vi "Plots_testing.vi"() -> ()   [LabVIEW 2016]
uses:
  <vilib>/Heliosphere Research LLC/Advanced Plotting Toolkit/api_plotting/Histogram2DProperties.ctl
  <vilib>/Heliosphere Research LLC/Advanced Plotting Toolkit/properties/Colormap.ctl
  <vilib>/Heliosphere Research LLC/Advanced Plotting Toolkit/properties/Colormap_Map.ctl
  <vilib>/Heliosphere Research LLC/Advanced Plotting Toolkit/properties/Colormap_Scaling.ctl
  <vilib>/Heliosphere Research LLC/Advanced Plotting Toolkit/properties/Display.ctl
  <vilib>/Heliosphere Research LLC/Advanced Plotting Toolkit/api_core/NewPlotType.ctl
  <vilib>/Heliosphere Research LLC/Advanced Plotting Toolkit/api_plotting/ArrayViewProperties.ctl
  SubVi's/SW_Globals.vi
  <vilib>/Heliosphere Research LLC/Advanced Plotting Toolkit/api_plotting/Histogram2D_Automatic.vi
  <vilib>/Heliosphere Research LLC/Advanced Plotting Toolkit/Advanced Plotting Toolkit.lvlib
panel:
  out "Picture 2":picture
  in  "Properties":T1={"Normalize"=FALSE, "Colormap"={"Map"=enum."Automatic", "Value Min"=nan, "Value Max"=nan, "Scaling"=enum."Default", "Reverse"=FALSE}, "Display"={"Alpha"=nan, "Z Order"=nan}}
  out "Count":u32[](array[numeric])
  out "X coords":i32[](array[numeric])
  out "Y coords":i32[](array[numeric])
  out "Picture":picture
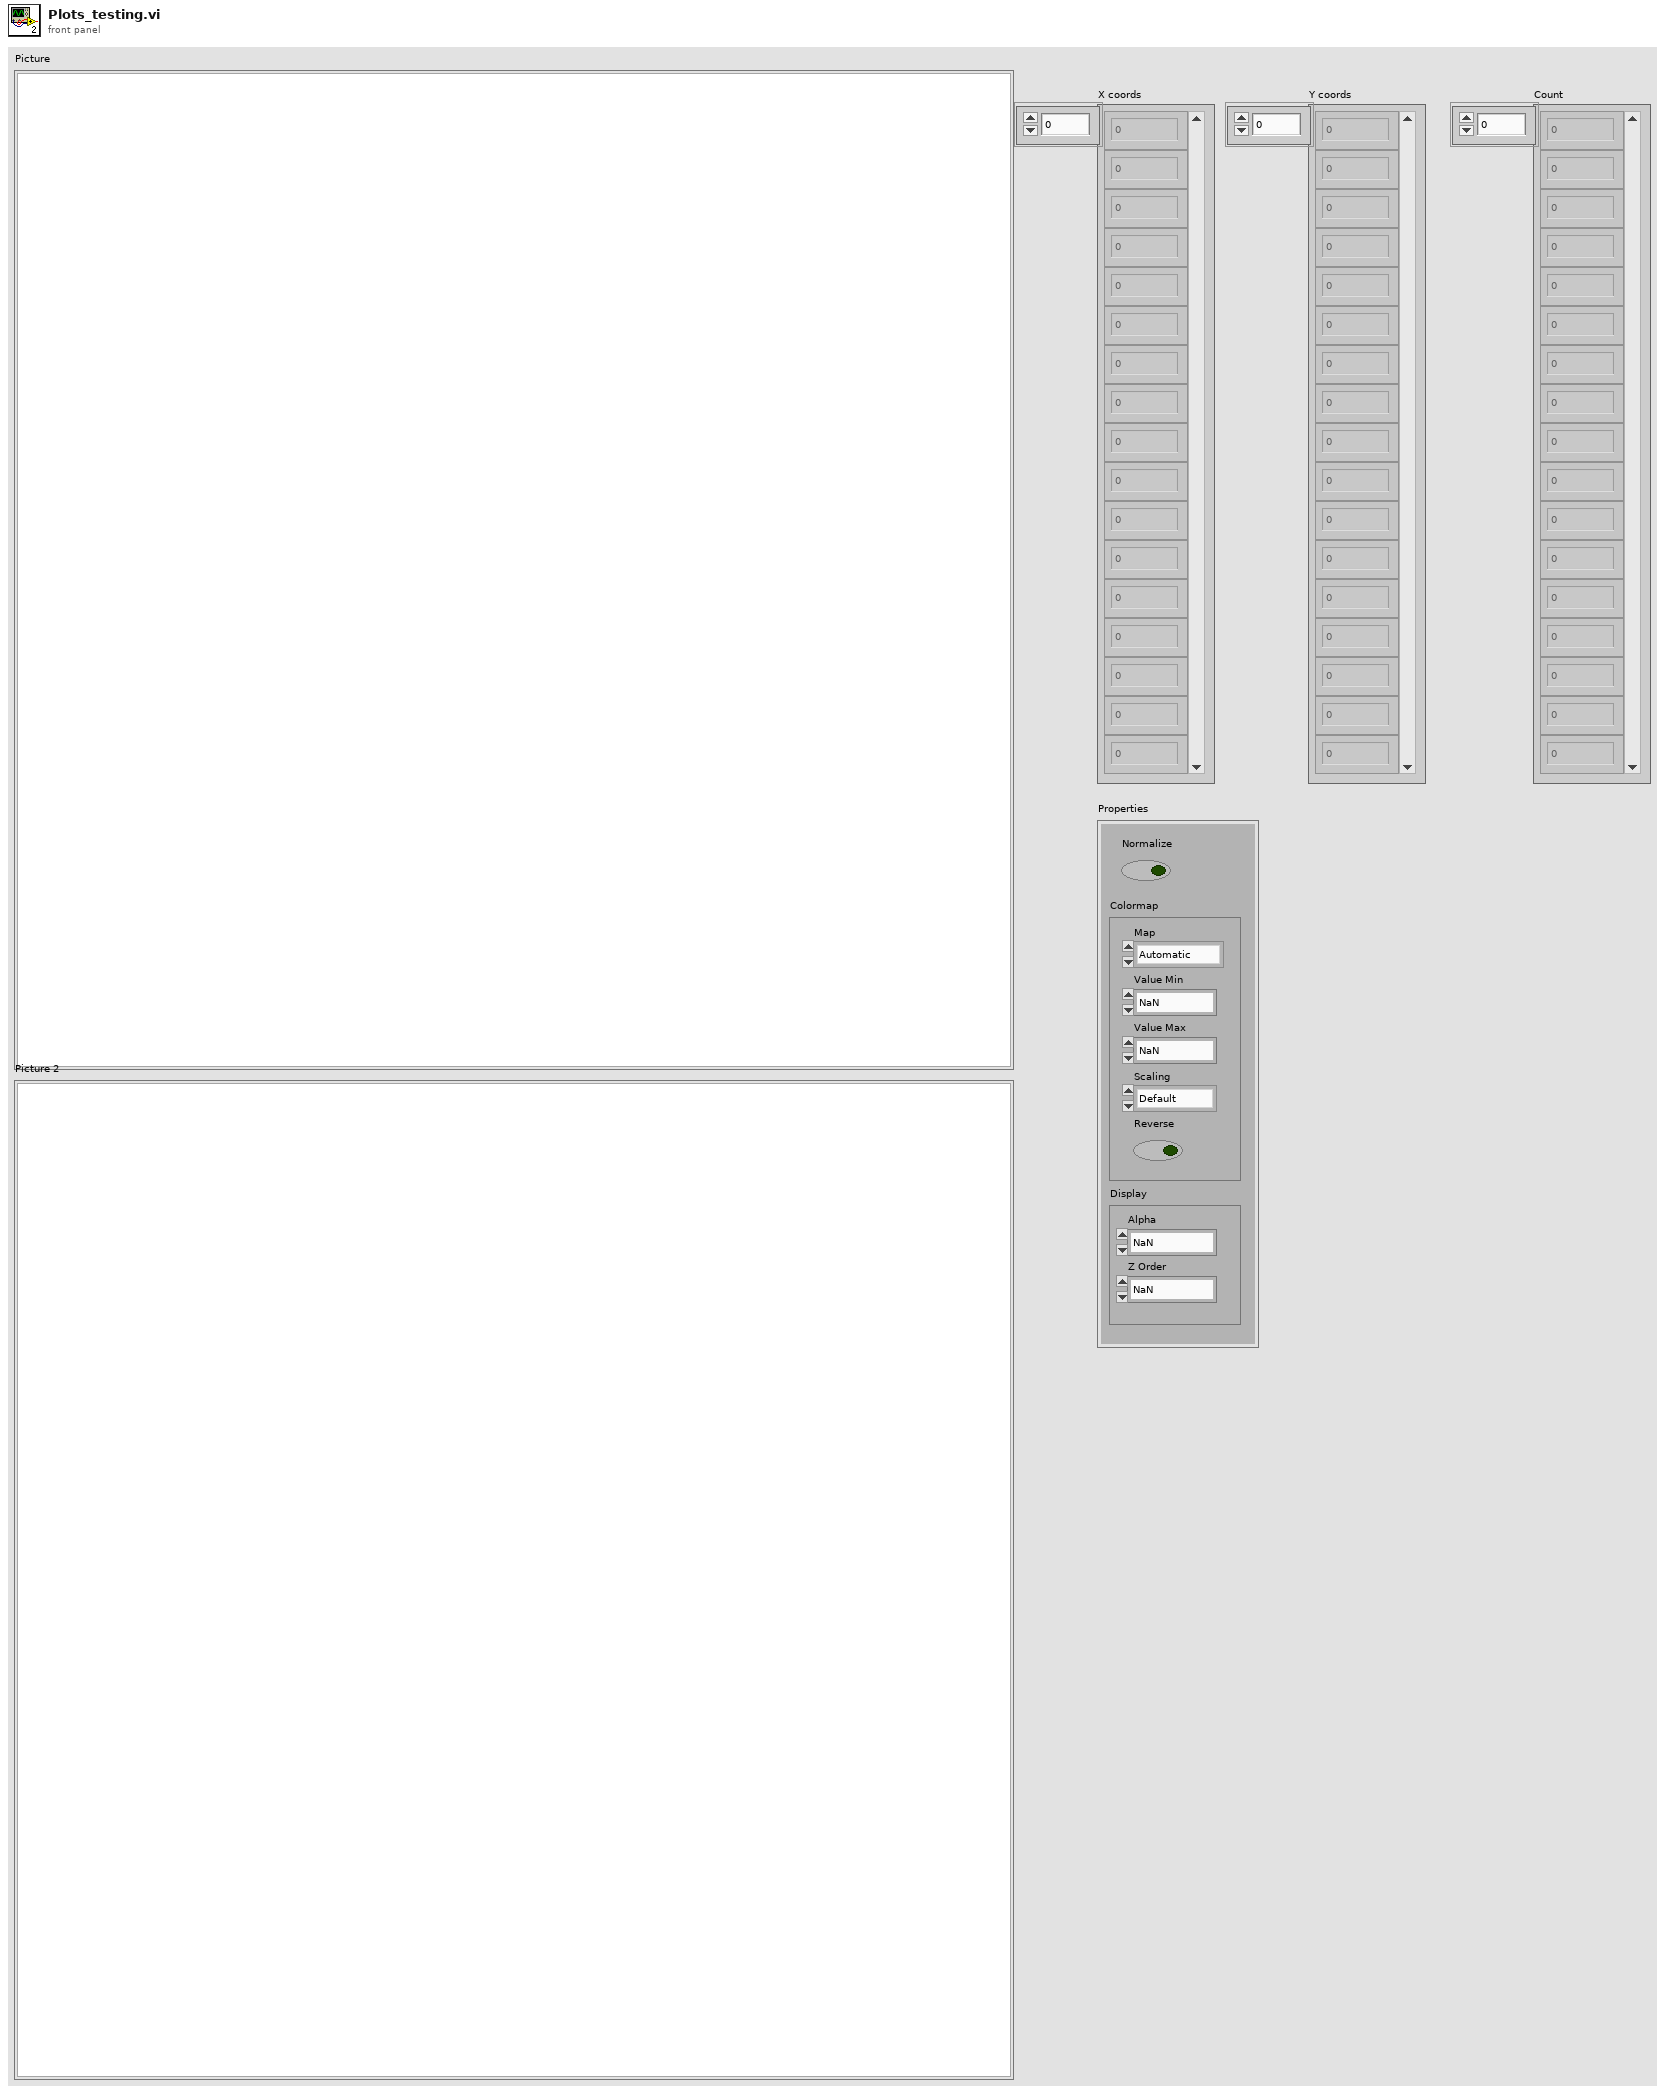
[diagram p1: front panel]
types:
  T1 = typedef "Advanced Plotting Toolkit.lvlib/Histogram2DProperties.ctl" = cluster{"Normalize":bool, "Colormap":T2, "Display":T5}
  T2 = typedef "Advanced Plotting Toolkit.lvlib/Colormap.ctl" = cluster{"Map":T3, "Value Min":dbl, "Value Max":dbl, "Scaling":T4, "Reverse":bool}
  T3 = typedef "Advanced Plotting Toolkit.lvlib/Colormap_Map.ctl" = enum16{"Automatic", "Rainbow", "Hot and Cold", "White-Black", "White-Blue", "White-Green", "White-Red", "Fire", "Water", "Earth", "Air", "Pastel", "Banded", "Stepped"}
  T4 = typedef "Advanced Plotting Toolkit.lvlib/Colormap_Scaling.ctl" = enum16{"Default"}
  T5 = typedef "Advanced Plotting Toolkit.lvlib/Display.ctl" = cluster{"Alpha":dbl, "Z Order":dbl}
  T6 = typedef "Advanced Plotting Toolkit.lvlib/ArrayViewProperties.ctl" = cluster{"Colormap":T2, "Display":T5}
  T7 = typedef "Advanced Plotting Toolkit.lvlib/NewPlotType.ctl" = enum16{"Rectangular Axes", "Polar Axes"}
  T8 = typedef "Advanced Plotting Toolkit.lvlib/PlotID.ctl" = i32
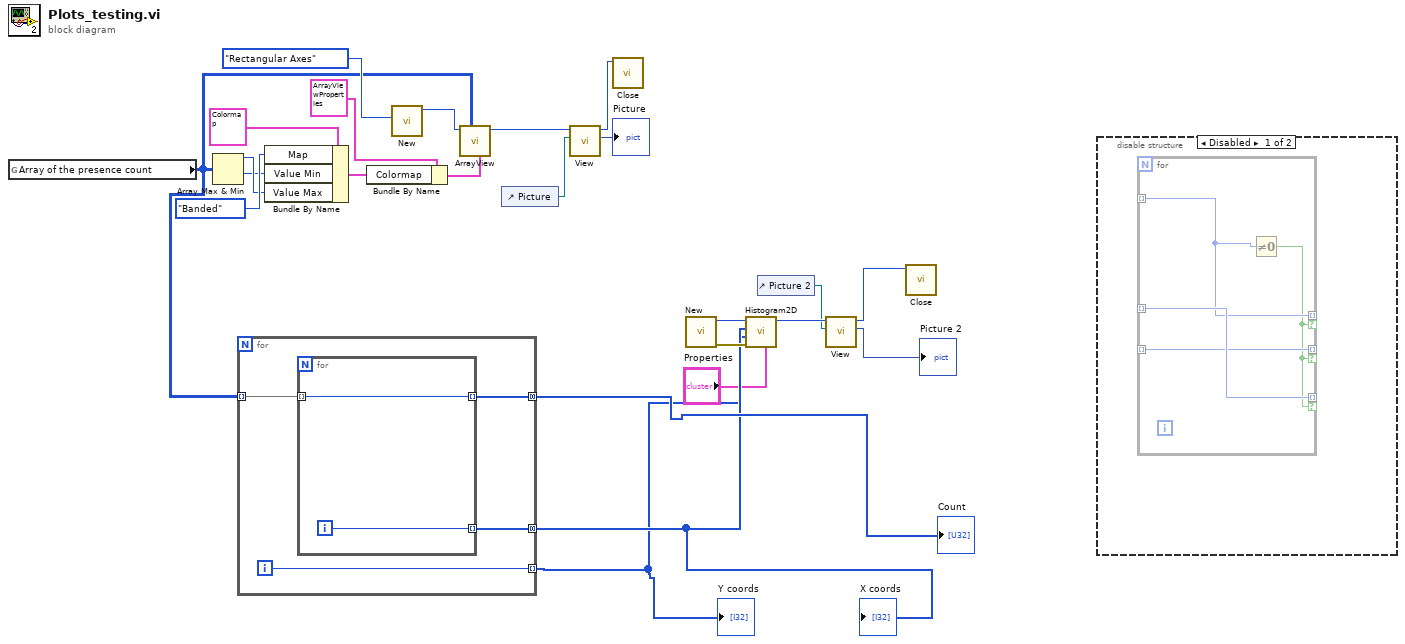
[diagram p0: block diagram]
diagram:
  n1 = global read "SW_Globals.vi" "Array of the presence count"() -> (w12:u32[][])
  n2 = Array Max & Min(array=w12) -> (max value=w14:u32, min value=w13:u32)  [unwired: 2 out]
  n3 = for {
    tunnel: w12 -> [w28] mode=indexing
    tunnel: [w27] -> w6 mode=indexing
    tunnel: [w26] -> w7 mode=concatenating
    tunnel: [w25] -> w10 mode=concatenating
    i -> [w27]
    n4 = for {
      tunnel: w28 -> [w29] mode=indexing
      tunnel: [w30] -> w26 mode=indexing
      tunnel: [w29] -> w25 mode=indexing
      i -> [w30]
    }
  }
  "Y coords" <- w6
  "X coords" <- w7
  "Count" <- w10
  n5 = Bundle By Name(cluster=T2 {"Map"=enum."Automatic", "Value Min"=nan, "Value Max"=nan, "Scaling"=enum."Default", "Reverse"=FALSE} ("Colormap"), "Map"=Colormap_Map."Banded", "Value Min"=w13, "Value Max"=w14) -> (w16:T2)
  n6 = Bundle By Name(cluster=T6 {"Colormap"={"Map"=enum."Automatic", "Value Min"=nan, "Value Max"=nan, "Scaling"=enum."Default", "Reverse"=FALSE}, "Display"={"Alpha"=nan, "Z Order"=nan}} ("Properties"), "Colormap"=w16) -> (w18:T6)
  n7 = call <vilib>:"New.vi"("Plot Type"=NewPlotType."Rectangular Axes") -> ("Plot ID"=w23:T8)  [unwired: 9 in, 1 out]
  n8 = call <vilib>:"ArrayView.vi"("Properties"=w18, "Data"=w12, "Plot ID"=w23) -> ("Plot ID Out"=w11:T8)  [unwired: 7 in, 1 out]
  n9 = control-ref of="Picture"() -> (w20:refnum<vi>)
  n10 = call <vilib>:"View.vi"("Ref for Sizing"=w20, "Plot ID"=w11) -> ("Picture"=→"Picture":picture, "Plot ID Out"=w21:T8)  [unwired: 7 in, 1 out]
  n11 = call <vilib>:"Close.vi"("Plot ID"=w21) -> ()  [unwired: 10 in, 1 out]
  n12 = call <vilib>:"New.vi"() -> ("error out"=w9:errorcluster, "Plot ID"=w8:T8)  [unwired: 10 in]
  n13 = call-poly <vilib>:"Histogram2D.vi"("Properties"="Properties", "error in (no error)"=w9, "Y Data"=w6, "X Data"=w7, "Plot ID"=w8) -> ("Plot ID Out"=w4:T8)  [unwired: 5 in, 1 out]
  n14 = control-ref of="Picture 2"() -> (w3:refnum<vi>)
  n15 = call <vilib>:"View.vi"("Ref for Sizing"=w3, "Plot ID"=w4) -> ("Picture"=→"Picture 2":picture, "Plot ID Out"=w2:T8)  [unwired: 7 in, 1 out]
  n16 = call <vilib>:"Close.vi"("Plot ID"=w2) -> ()  [unwired: 10 in, 1 out]
  n17 = disable-structure shown="Disabled" {
    frame Disabled {
      n18 = for {
        tunnel: _ -> [w32] mode=indexing
        tunnel: _ -> [w34] mode=indexing
        tunnel: _ -> [w33] mode=indexing
        tunnel: [w32] -> _ mode=indexing if=w31
        tunnel: [w34] -> _ mode=indexing if=w31
        tunnel: [w33] -> _ mode=indexing if=w31
        n19 = Not Equal To 0?(x=w32) -> (x != 0?=w31:bool)
      }
    }
    frame Enabled {
    }
  }
